vi "Get Distance From Row Positions 1D Array.vi"(1 "Row":dbl, 2 "DistanceArray":dbl[](array[numeric])) -> (0 "Value":dbl)   [LabVIEW 2014, in "Position.lvclass"]
uses:
  Position.lvclass
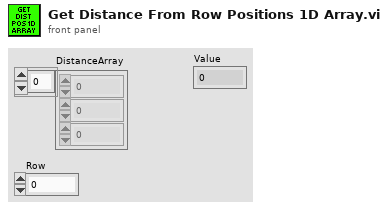
[diagram p1: front panel]
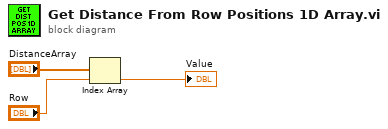
[diagram p0: block diagram]
diagram:
  n1 = Index Array(array="DistanceArray", index="Row") -> (element=→"Value":dbl)
